vi "Initialize2.vi"(6 "Files":T1, 8 "Status/Errors in":refnum<vi>, 9 "Control Parameters [] in":T25[](array[typedef]) {"Aux Byte Value" format="%02x"; "Max Real Value" format="%#_6e"; "Min Real Value" format="%#_6e"; "dReal/dByte" format="%#_6e"; "Byte Value" format="%02x"; "Identifier" format="%02x"}, 10 "Mode":T4={"Mode"=enum."Dialog", "Expert?"=FALSE, "Dialog?"=FALSE}) -> (0 "Status/Errors out":refnum<vi>, 1 "Control Parameters [] out":T25[](array[typedef]) {"Aux Byte Value" format="%02x"; "Max Real Value" format="%#_6e"; "Min Real Value" format="%#_6e"; "dReal/dByte" format="%#_6e"; "Byte Value" format="%02x"; "Identifier" format="%02x"}, 2 "Parameters":T3={"Mode"={"Mode"=enum."Dialog", "Expert?"=FALSE, "Dialog?"=FALSE}, "Stop loop"={"Settings changed?"=FALSE, "Stop?"=refnum}, "Send message"={"Send mode"=enum."Get parameters", "Set parameter list"=0, "Get parameter list"=0, "Reset device"=0, "Length set settings message"=0, "Reset buttons?"=FALSE, "Reset Master?"=enum."General"}, "Write settings"={"Options"=enum."File 1"}, "Read bytes"={"Max bytes read"=0, "Max bytes reached?"=FALSE}, "Settings state"={"MAS locked?"=refnum, "SLV locked?"=refnum}, "Button refs"={"Stop program"=refnum, "Save settings"=refnum, "DAQ mode"=refnum, "Reset settings"=refnum, "Apply settings"=refnum, "Reset MAS"=refnum, "Reset SLV"=refnum, "Local DBase?"=refnum, "Last value DBase"=FALSE, "Database"=refnum, "Calibration"=refnum, "Save settings 2"=refnum}, "Process messages"={"Process message mode"=enum."Error", "Slave data?"=FALSE, "Length get settings message"=0, "Delta time"=0.0, "Data_Filter"={"Filter_Data"=FALSE, "Use_Thresh"=FALSE, "Reduce data?"=FALSE}, "Time_difference_stack"=[], "Starting sec"=0, "Ending sec"=0, "Ending sec 2"=0, "MAS_Page_Thresh"=refnum, "SLV_Page_Thresh"=refnum, "Database"=refnum}, "Data storage"={"DB connection"={"connection reference"=refnum, "Connected?"=refnum, "ODBC Name"=""}, "Data storage condition"={"Database?"=FALSE}, "Detector number"=0, "# Messages to send"=0, "Database"=refnum, "Password"="", "Last error message"={"Last error message time stamp"={"Seconds"=0, "Minutes"=0, "Hours"=0, "Day"=0, "Month"=0, "Year"=0}, "Last error log"="", "Last error message"=""}, "Status_id"=refnum, "Hardware"=enum."None"}, "Update screen"={"Detector number"=0, "Hardware"=enum."None"}, "Alignment parameters"=refnum, "Timer parameters"=refnum, "Files"={"Path config file"=path "", "Path def. ini file"=path "", "Path ini file 1"=path "", "Path ini file 2"=path "", "Path RBF file"=path ""}, "Status_id"=refnum, "Time difference"=refnum, "Satellites"=refnum, "Calibration"={"GEN_Page_Calibrate"=refnum, "MAS_Page_Gain"=refnum, "MAS_Page_Offset"=refnum, "SLV_Page_Gain"=refnum, "SLV_Page_Offset"=refnum, "MAS_Page_Common"=refnum, "SLV_Page_Common"=refnum}, "Page Statistics 2"=refnum, "Page Statistics"=refnum} {"Update screen"."Detector number" format="%#.0f"; "Data storage"."Detector number" format="%#.0f"; "Read bytes"."Max bytes read" format="%#.0f"; "Send message"."Reset device" format="%x"; "Send message"."Get parameter list" format="%x"; "Send message"."Set parameter list" format="%x"}, 3 "Devices":T24, 4 "Queues":T2, 5 "Timer parameters out":refnum<vi>)   [LabVIEW 2010]
uses:
  Controls/Control_Parameters.ctl
  Controls/Master.ctl
  Controls/Devices.ctl
  Controls/Timer_Parameters.ctl
  Controls/Mode.ctl
  Controls/Parameters.ctl
  Controls/Stop_Loop.ctl
  Controls/Send_Message.ctl
  Controls/Send_Message_Mode.ctl
  Controls/Write_Settings.ctl
  Controls/Write_Settings_Options.ctl
  Controls/Read_Bytes.ctl
  Controls/Settings_State.ctl
  Controls/Button_Refs.ctl
  Controls/Process_Messages.ctl
  Controls/Process_Message_Mode.ctl
  Controls/Data_Storage.ctl
  Controls/DB_Connection.ctl
  database/Connection.llb/Conn ObjectReference.ctl
  Controls/Data_Storage_Condition.ctl
  Controls/GPS_Timestamp.ctl
  Controls/Update_Screen.ctl
  Controls/Files.ctl
  Controls/Page_Calibration.ctl
  Controls/Queues.ctl
  Controls/One_Second.ctl
panel:
  out "Timer parameters":T23={"current time (ms)"=0, "time (ms) screen updated"=0, "time (ms) controls locked"=0, "time (ms) last device check"=0, "time (ms) last data MAS"=0, "time (ms) last data SLV"=0, "time (ms) bad status MAS"=0, "time (ms) bad status SLV"=0, "time (ms) clock error updated"=0, "time delay screen update (ms)"=0, "time delay controls (ms)"=0, "time delay device check (ms)"=5000, "time until MAS status bad (ms)"=5000, "time until SLV status bad (ms)"=5000, "time until MAS connection bad (ms)"=5000, "time until SLV connection bad (ms)"=10000, "time delay clock error update (ms)"=600000}
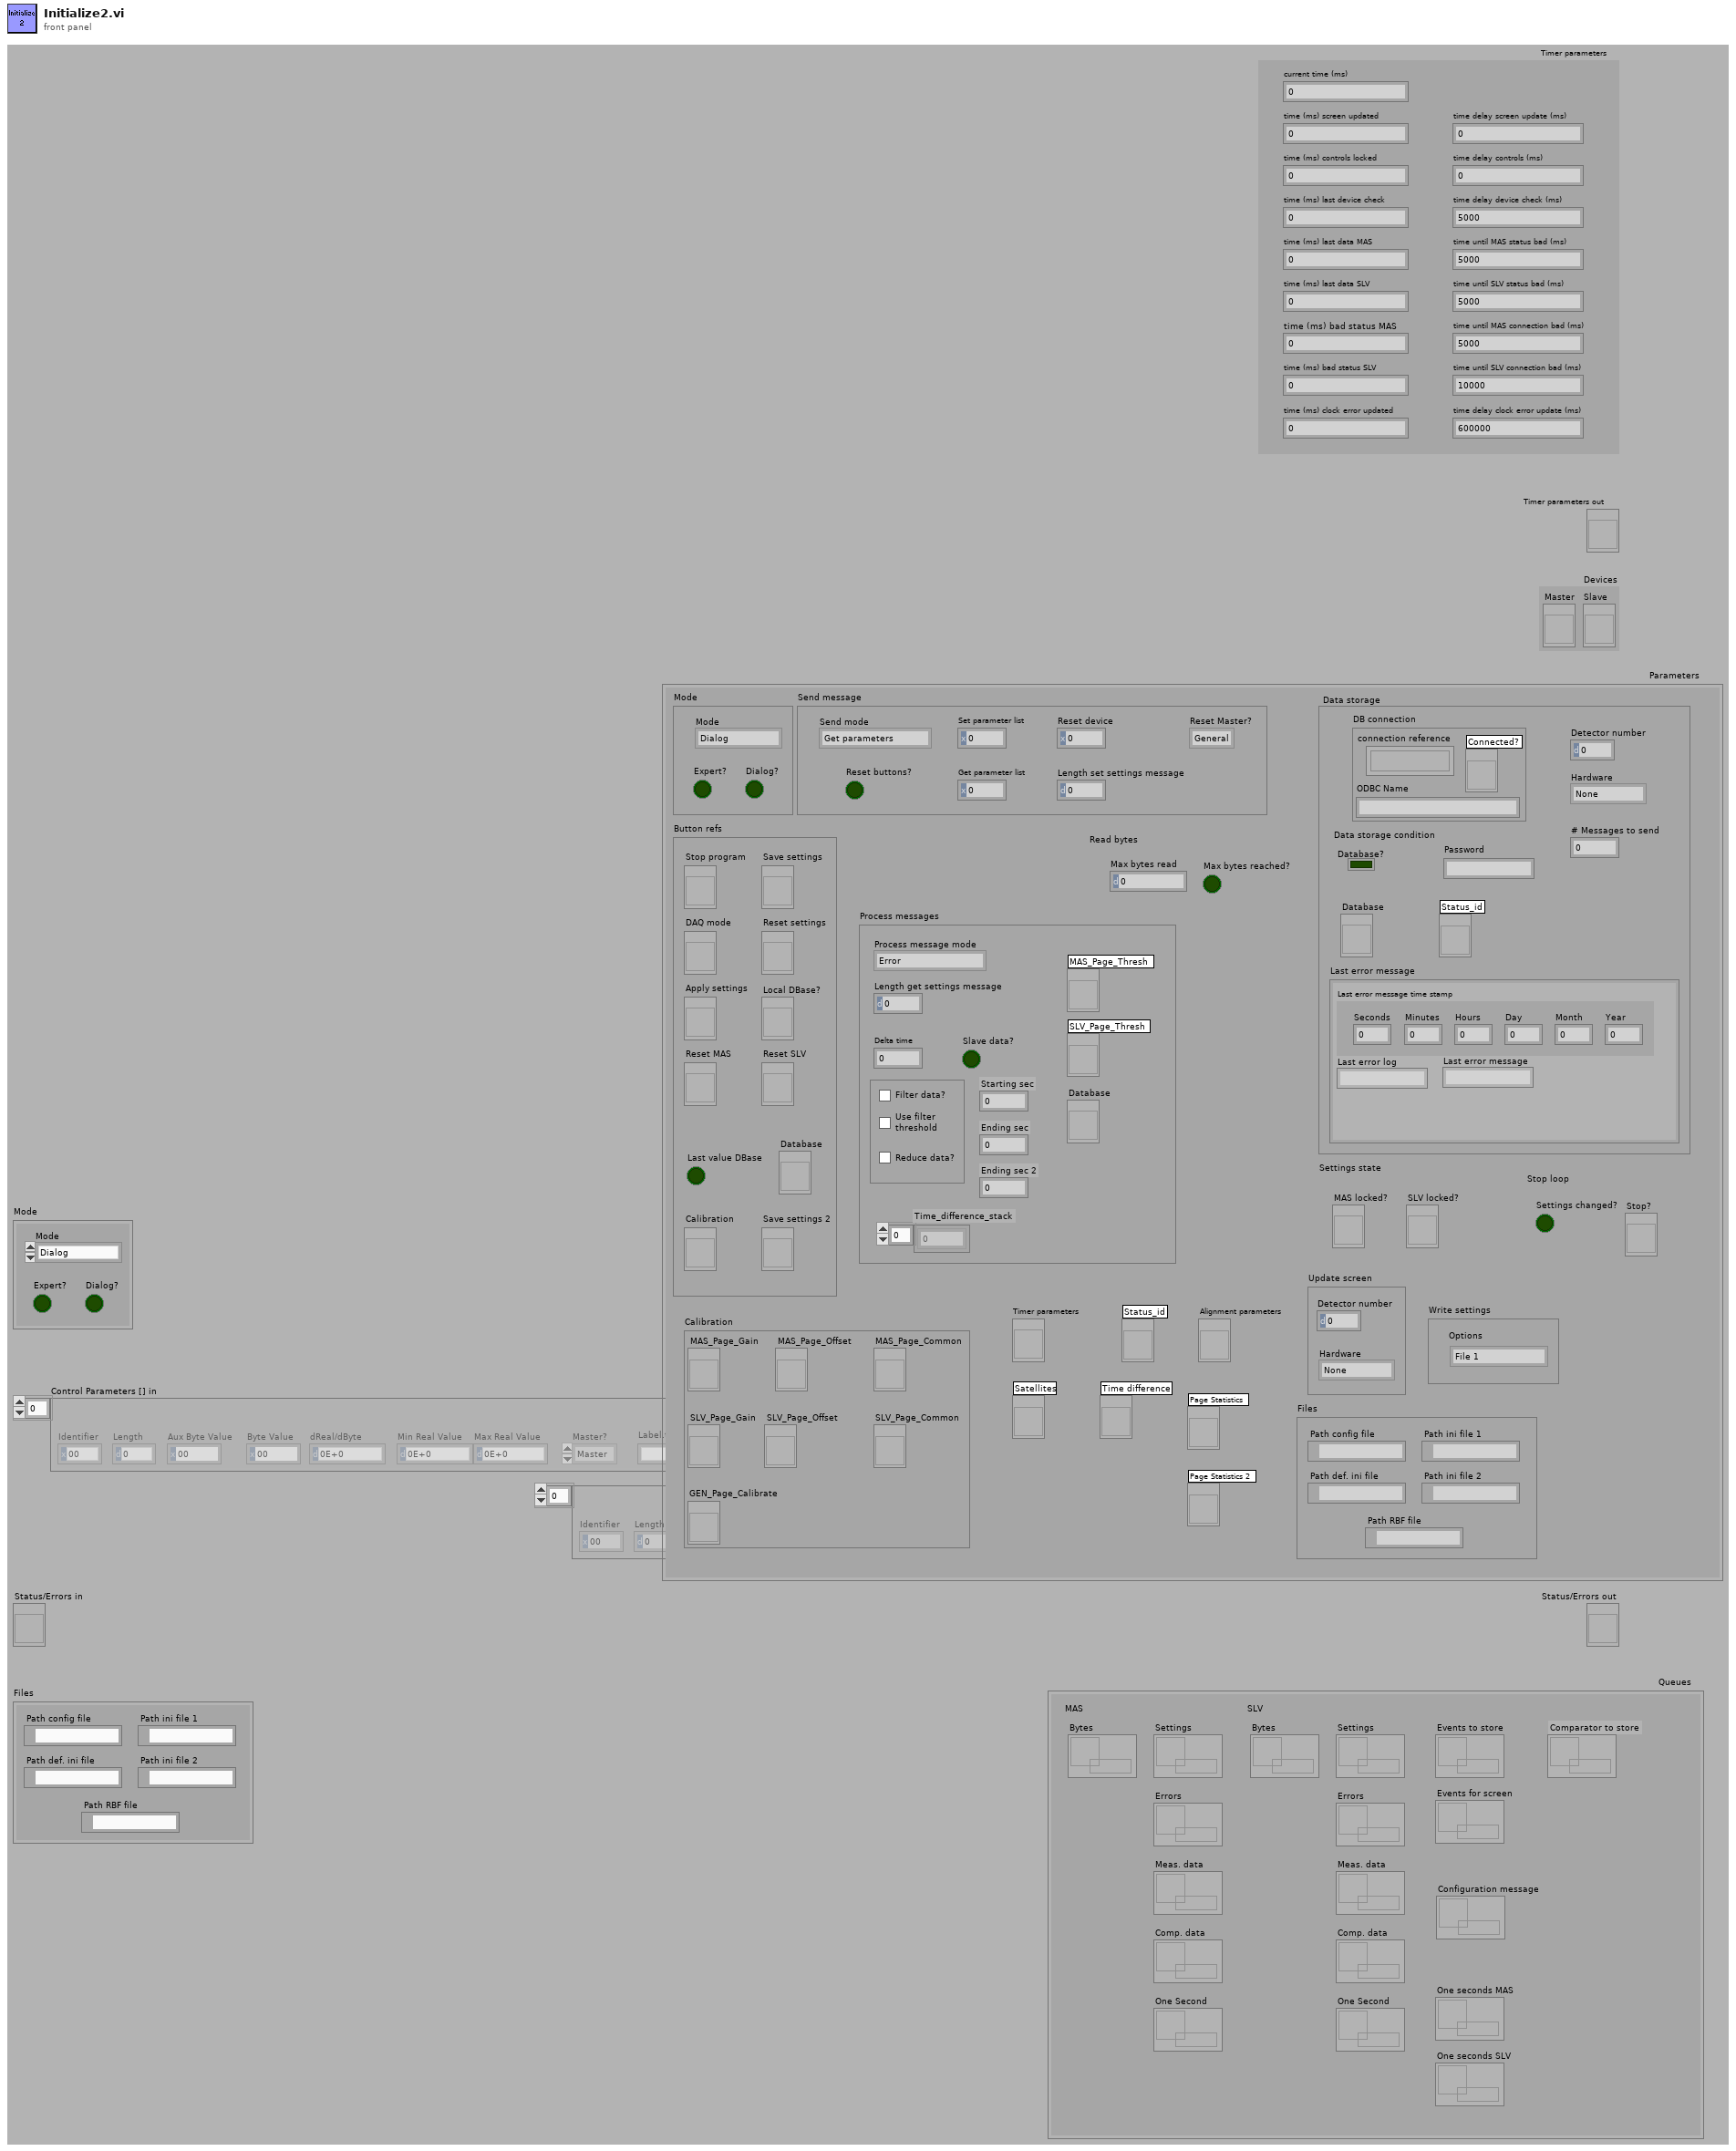
[diagram p1: front panel]
types:
  T1 = typedef "Files.ctl" = cluster{"Path config file":path, "Path def. ini file":path, "Path ini file 1":path, "Path ini file 2":path, "Path RBF file":path}
  T2 = typedef "Queues.ctl" = cluster{"MAS":cluster{"Bytes":refnum<queue>, "Settings":refnum<queue>, "Errors":refnum<queue>, "Meas. data":refnum<queue>, "One Second":refnum<queue>, "Comp. data":refnum<queue>}, "SLV":cluster{"Bytes":refnum<queue>, "Settings":refnum<queue>, "Errors":refnum<queue>, "Meas. data":refnum<queue>, "One Second":refnum<queue>, "Comp. data":refnum<queue>}, "Events to store":refnum<queue>, "Events for screen":refnum<queue>, "One seconds MAS":refnum<queue>, "One seconds SLV":refnum<queue>, "Configuration message":refnum<queue>, "Comparator to store":refnum<queue>}
  T3 = typedef "Parameters.ctl" = cluster{"Mode":T4, "Stop loop":T5, "Send message":T6, "Write settings":T9, "Read bytes":T11, "Settings state":T12, "Button refs":T13, "Process messages":T14, "Data storage":T16, "Update screen":T21, "Alignment parameters":refnum<vi>, "Timer parameters":refnum<vi>, "Files":T1, "Status_id":refnum<vi>, "Time difference":refnum<vi>, "Satellites":refnum<vi>, "Calibration":T22, "Page Statistics 2":refnum<vi>, "Page Statistics":refnum<vi>}
  T4 = typedef "Mode.ctl" = cluster{"Mode":enum8{"Stop", "Dialog", "Hisparc II", "Hisparc II DAQ", "Alignment"}, "Expert?":bool, "Dialog?":bool}
  T5 = typedef "Stop_Loop.ctl" = cluster{"Settings changed?":bool, "Stop?":refnum<vi>}
  T6 = typedef "Send_Message.ctl" = cluster{"Send mode":T7, "Set parameter list":u8, "Get parameter list":u8, "Reset device":u8, "Length set settings message":i32, "Reset buttons?":bool, "Reset Master?":T8}
  T7 = typedef "Send_Message_Mode.ctl" = enum16{"Get parameters", "Set parameters", "From front panel", "From parameters", "Reset device", "Alignment"}
  T8 = typedef "Master.ctl" = enum16{"Master", "Slave", "General"}
  T9 = typedef "Write_Settings.ctl" = cluster{"Options":T10}
  T10 = typedef "Write_Settings_Options.ctl" = enum16{"File 1", "File 2", "Alignment", "Reset"}
  T11 = typedef "Read_Bytes.ctl" = cluster{"Max bytes read":u32, "Max bytes reached?":bool}
  T12 = typedef "Settings_State.ctl" = cluster{"MAS locked?":refnum<vi>, "SLV locked?":refnum<vi>}
  T13 = typedef "Button_Refs.ctl" = cluster{"Stop program":refnum<vi>, "Save settings":refnum<vi>, "DAQ mode":refnum<vi>, "Reset settings":refnum<vi>, "Apply settings":refnum<vi>, "Reset MAS":refnum<vi>, "Reset SLV":refnum<vi>, "Local DBase?":refnum<vi>, "Last value DBase":bool, "Database":refnum<vi>, "Calibration":refnum<vi>, "Save settings 2":refnum<vi>}
  T14 = typedef "Process_Messages.ctl" = cluster{"Process message mode":T15, "Slave data?":bool, "Length get settings message":i32, "Delta time":dbl, "Data_Filter":cluster{"Filter_Data":bool, "Use_Thresh":bool, "Reduce data?":bool}, "Time_difference_stack":u64[], "Starting sec":u64, "Ending sec":u64, "Ending sec 2":u64, "MAS_Page_Thresh":refnum<vi>, "SLV_Page_Thresh":refnum<vi>, "Database":refnum<vi>}
  T15 = typedef "Process_Message_Mode.ctl" = enum16{"Error", "Measurement data", "Comparator data", "One Second"}
  T16 = typedef "Data_Storage.ctl" = cluster{"DB connection":T17, "Data storage condition":T19, "Detector number":u16, "# Messages to send":i32, "Database":refnum<vi>, "Password":string, "Last error message":cluster{"Last error message time stamp":T20, "Last error log":string, "Last error message":string}, "Status_id":refnum<vi>, "Hardware":enum8{"None", "HiSPARC I", "HiSPARC II", "HiSPARC III", "Unknown"}}
  T17 = typedef "DB_Connection.ctl" = cluster{"connection reference":T18, "Connected?":refnum<vi>, "ODBC Name":string}
  T18 = typedef "Conn ObjectReference.ctl" = refnum<k1>
  T19 = typedef "Data_Storage_Condition.ctl" = cluster{"Database?":bool}
  T20 = typedef "GPS_Timestamp.ctl" = cluster{"Seconds":u8, "Minutes":u8, "Hours":u8, "Day":u8, "Month":u8, "Year":u16}
  T21 = typedef "Update_Screen.ctl" = cluster{"Detector number":u16, "Hardware":enum8{"None", "HiSPARC I", "HiSPARC II", "HiSPARC III", "Unknown"}}
  T22 = typedef "Page_Calibration.ctl" = cluster{"GEN_Page_Calibrate":refnum<vi>, "MAS_Page_Gain":refnum<vi>, "MAS_Page_Offset":refnum<vi>, "SLV_Page_Gain":refnum<vi>, "SLV_Page_Offset":refnum<vi>, "MAS_Page_Common":refnum<vi>, "SLV_Page_Common":refnum<vi>}
  T23 = typedef "Timer_Parameters.ctl" = cluster{"current time (ms)":u32, "time (ms) screen updated":u32, "time (ms) controls locked":u32, "time (ms) last device check":u32, "time (ms) last data MAS":u32, "time (ms) last data SLV":u32, "time (ms) bad status MAS":u32, "time (ms) bad status SLV":u32, "time (ms) clock error updated":u32, "time delay screen update (ms)":u32, "time delay controls (ms)":u32, "time delay device check (ms)":u32, "time until MAS status bad (ms)":u32, "time until SLV status bad (ms)":u32, "time until MAS connection bad (ms)":u32, "time until SLV connection bad (ms)":u32, "time delay clock error update (ms)":u32}
  T24 = typedef "Devices.ctl" = cluster{"Master":refnum<vi>, "Slave":refnum<vi>}
  T25 = typedef "Control_Parameters.ctl" = cluster{"Identifier":u8, "Length":u16, "Byte Value":u32, "dReal/dByte":dbl, "Min Real Value":dbl, "Max Real Value":dbl, "Master?":T8, "Label.text":string, "Description":string, "Refnum":refnum<vi>, "Aux Byte Value":u32}
  T26 = typedef "Main_Parameters.ctl" = cluster{"Mode":T4, "Stop loop":T5, "Send message":T6, "Write settings":T9, "Settings state":T12, "Button refs":T13, "Update screen":T21, "Files":T1, "DB connection":T17, "Status_id":refnum<vi>, "Time difference":refnum<vi>, "Satellites":refnum<vi>, "Alignment parameters":refnum<vi>, "Page Statistics 2":refnum<vi>, "Database":refnum<vi>, "Page Statistics":refnum<vi>}
  T27 = enum8{"Stop", "Dialog", "Hisparc II", "Hisparc II DAQ", "Alignment"}
  T28 = enum16{"Only front panel", "Only buttons", "Both", "Invisible"}
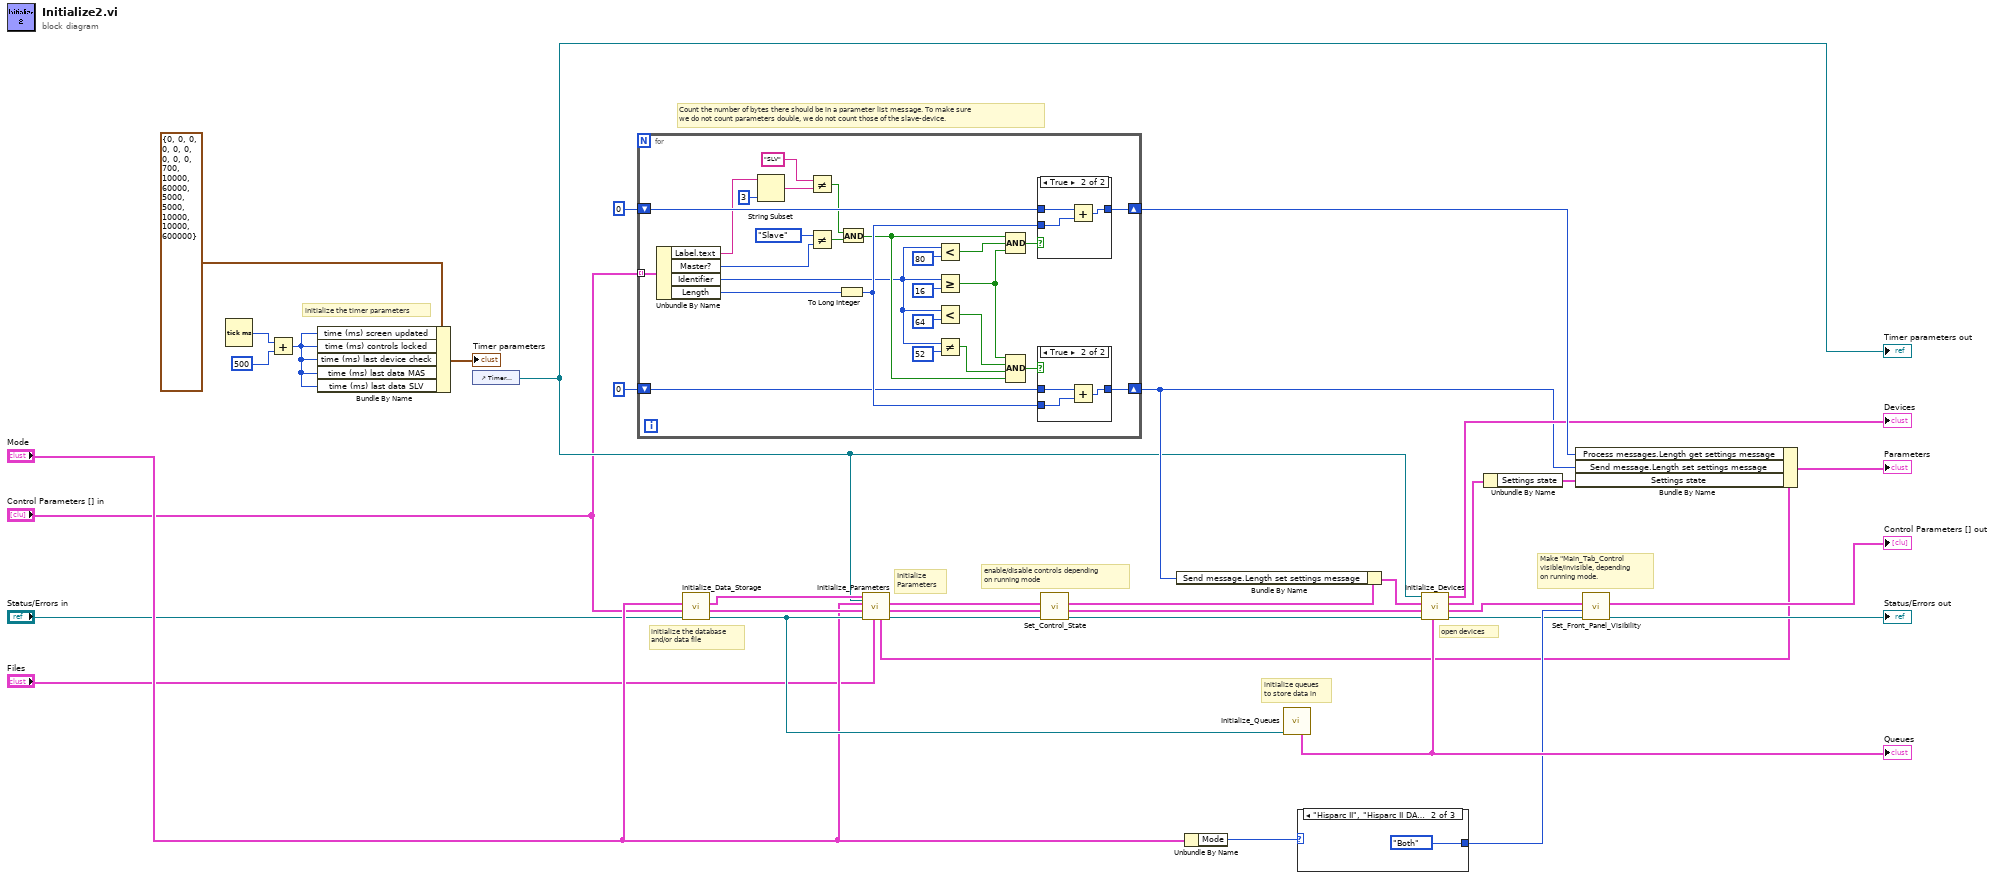
[diagram p0: block diagram]
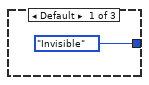
[diagram p2: hidden frame]
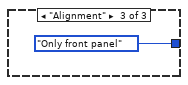
[diagram p3: hidden frame]
diagram:
  # "enable/disable controls depending\non running mode"
  # "initialize queues\nto store data in"
  # "Initialize\nParameters"
  # "Make \"Main_Tab_Control\nvisible/invisible, depending\non running mode."
  # "initialize the database\nand/or data file"
  # "Count the number of bytes there should be in a parameter list message. To make sure\nwe do not count parameters double, we do not count those of the slave-device."
  # "initialize the timer parameters"
  # "open devices"
  n1 = Tick Count (ms)() -> (millisecond timer value=w23:u32)
  n2 = Add(x=w23, y=u32 500) -> (x+y=w18:u32)
  n3 = Bundle By Name(cluster=T23 {"current time (ms)"=0, "time (ms) screen updated"=0, "time (ms) controls locked"=0, "time (ms) last device check"=0, "time (ms) last data MAS"=0, "time (ms) last data SLV"=0, "time (ms) bad status MAS"=0, "time (ms) bad status SLV"=0, "time (ms) clock error updated"=0, "time delay screen update (ms)"=700, "time delay controls (ms)"=10000, "time delay device check (ms)"=60000, "time until MAS status bad (ms)"=5000, "time until SLV status bad (ms)"=5000, "time until MAS connection bad (ms)"=10000, "time until SLV connection bad (ms)"=10000, "time delay clock error update (ms)"=600000} ("Timer parameters out"), "time (ms) screen updated"=w18, "time (ms) controls locked"=w18, "time (ms) last device check"=w18, "time (ms) last data MAS"=w18, "time (ms) last data SLV"=w18) -> (→"Timer parameters":T23)
  n4 = control-ref of="Timer parameters"() -> (w15:refnum<vi>)
  "Timer parameters out" <- w15
  n5 = for {
    tunnel: "Control Parameters [] in" -> [w58] mode=indexing
    shift-right: [w59] -> w32
    shift-left: 0 -> [w60]
    shift-right: [w51] -> w20
    shift-left: 0 -> [w50]
    n6 = Unbundle By Name(w58) -> ("Label.text"=w49:string, "Master?"=w63:T8, "Identifier"=w41:u8, "Length"=w53:u16)
    n7 = String Subset(string=w49, length (rest)=3 ("length (rest)")) -> (substring=w47:string)  [unwired: 1 out]
    n8 = Not Equal?(x="SLV", y=w47) -> (x != y?=w44:bool)
    n9 = Not Equal?(x=Master."Slave" ("Master?"), y=w63) -> (x != y?=w45:bool)
    n10 = To Long Integer(number=w53) -> (32bit integer=w52:i32)
    n11 = And(x=w44, y=w45) -> (x .and. y?=w43:bool)
    n12 = Less?(x=w41, y=u8 80) -> (x < y?=w39:bool)
    n13 = Greater Or Equal?(x=w41, y=u8 16) -> (x >= y?=w38:bool)
    n14 = Less?(x=w41, y=u8 64) -> (x < y?=w37:bool)
    n15 = Not Equal?(x=w41, y=u8 52) -> (x != y?=w40:bool)
    n16 = Compound Arithmetic op=AND(w43, w39, w38) -> (w61:bool)
    n17 = Compound Arithmetic op=AND(w38, w37, w40, w43) -> (w54:bool)
    n18 = case shown="True" w61 {
      tunnel: w52 -> [_ w71]
      tunnel: w60 -> [w68 w70]
      tunnel: [w68 w69] -> w59
      frame False {
      }
      frame True {
        n19 = Add(x=w70, y=w71) -> (x+y=w69:i32)
      }
    }
    n20 = case shown="True" w54 {
      tunnel: w52 -> [_ w67]
      tunnel: w50 -> [w64 w66]
      tunnel: [w64 w65] -> w51
      frame False {
      }
      frame True {
        n21 = Add(x=w66, y=w67) -> (x+y=w65:i32)
      }
    }
  }
  n22 = call "Initialize_Data_Storage.vi"("Status/Errors in"="Status/Errors in", "Control Parameters [] in"="Control Parameters [] in", "Mode"="Mode") -> ("Status/Errors out"=w25:refnum<vi>, "Control Parameters [] out"=w27:T25[], "Data storage"=w26:T16)  [unwired: 6 out]
  n23 = call "Initialize_Parameters.vi"("Files"="Files", "Timer parameters"=w15, "Status/Errors in"=w25, "Control parameters [] in"=w27, "Mode"="Mode", "Data storage"=w26) -> ("Status/Errors out"=w11:refnum<vi>, "Control parameters [] out"=w9:T25[], "Main parameters"=w7:T26, "Parameters"=w4:T3)  [unwired: 2 out]
  n24 = call "Set_Control_State.vi"("Status/Errors in"=w11, "Control Parameters [] in"=w9, "Main parameters in"=w7) -> ("Status/Errors out"=w10:refnum<vi>, "Control Parameters [] out"=w8:T25[], "Main parameters out"=w6:T26)  [unwired: 2 in, 4 out]
  n25 = Bundle By Name(cluster=w6, "Send message.Length set settings message"=w20) -> (w19:T26)
  n26 = Unbundle By Name("Mode") -> ("Mode"=w34:T27)
  n27 = call "Initialize_Queues.vi"("Status/Errors in"=w25) -> ("Queues"=w24:T2)  [unwired: 10 out]
  "Queues" <- w24
  n28 = case shown="\"Hisparc II\", \"Hisparc II DAQ\"" w34 {
    tunnel: [T28."Invisible" ("Visibility") T28."Both" ("Visibility") T28."Only front panel" ("Visibility")] -> w16
    frame Default {
    }
    frame "Hisparc II", "Hisparc II DAQ" {
    }
    frame "Alignment" {
    }
  }
  n29 = call "Initialize_Devices.vi"("Queues"=w24, "Status/Errors in"=w10, "Control Parameters [] in"=w8, "Main parameters in"=w19, "Timer parameters"=w15) -> ("Status/Errors out"=w12:refnum<vi>, "Control Parameters [] out"=w13:T25[], "Main parameters out"=w14:T26, "Devices"=→"Devices":T24)  [unwired: 1 in, 2 out]
  n30 = Unbundle By Name(w14) -> ("Settings state"=w28:T12)
  n31 = Bundle By Name(cluster=w4, "Process messages.Length get settings message"=w32, "Send message.Length set settings message"=w20, "Settings state"=w28) -> (→"Parameters":T3)
  n32 = call "Set_Front_Panel_Visibility.vi"("Status/Errors in"=w12, "Visibility"=w16, "Control Parameters [] in"=w13) -> ("Status/Errors out"=→"Status/Errors out":refnum<vi>, "Control Parameters [] out"=→"Control Parameters [] out":T25[])  [unwired: 7 out]
